vi "Intan_CreateBinaryFile.vi"() -> ()   [LabVIEW 2011]
panel:
  out "error out":errorcluster
  out "refnum out":refnum<file>
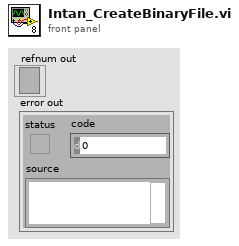
[diagram p1: front panel]
types:
  T1 = enum16{"open", "replace", "create", "open or create", "replace or create", "replace or create with confirmation"}
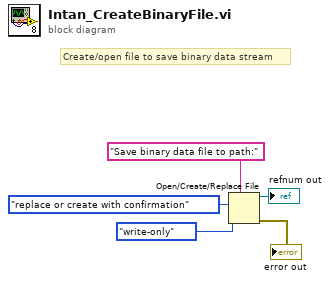
[diagram p0: block diagram]
diagram:
  # "Create/open file to save binary data stream"
  n1 = Open/Create/Replace File(prompt="Save binary data file to path:" ("prompt (Choose or enter file path)"), operation (0:open)=T1."replace or create with confirmation", access (0:read/write)=enum16{"read/write", "read-only", "write-only"}."write-only") -> (refnum out=→"refnum out":refnum<file>, error out=→"error out":errorcluster)  [unwired: 3 in, 1 out]
